vi "Version.vi"(8 "error in":errorcluster) -> (0 "error out":errorcluster, 3 "version":string)   [LabVIEW 2026, in "synnax_clib.lvlib" / "Synnax Client.lvclass"]
doc: "SYNNAX_EXPORT const char *synnax_client_version(void);"
uses:
  Synnax Client.lvclass
  Synnax Client.lvclass/Synnax Client.ctl
  synnax_clib.dll
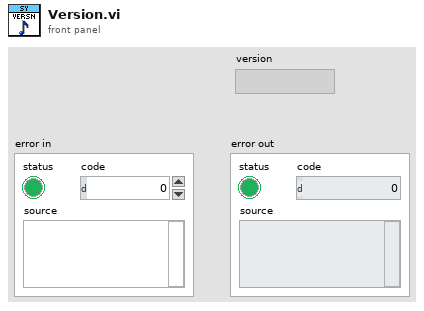
[diagram p1: front panel]
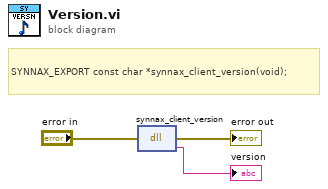
[diagram p0: block diagram]
diagram:
  # "SYNNAX_EXPORT const char *synnax_client_version(void);"
  n1 = dll-call lib="C/synnax/client/labview/synnax_clib.*" fn="synnax_client_version"(error in="error in") -> (error out=→"error out":errorcluster, →"version":string)  [unwired: 2 in, 1 out]
